vi "Test2.vi"   [LabVIEW 2011]
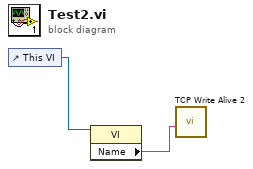
[diagram p0: block diagram]
diagram:
  n1 = control-ref of="This VI"() -> (w2:refnum<vi>)
  n2 = property class="VI"(reference=w2) -> ("Name"=w1:string)  [unwired: 1 in, 2 out]
  n3 = call "TCP Write Alive 2.vi"("Name"=w1) -> ()  [unwired: 11 in]
